vi "控制箱到引脚映射.vi"(1 "导通控制箱":string) -> (0 "导通引脚":string)   [LabVIEW 2020]
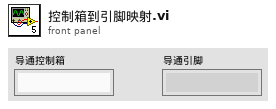
[diagram p1: front panel]
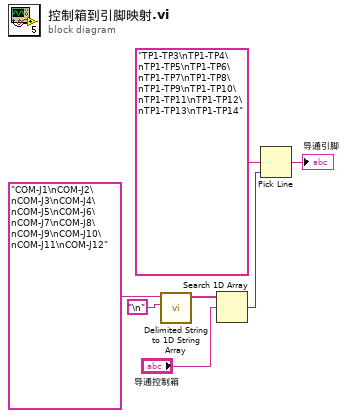
[diagram p0: block diagram]
diagram:
  n1 = call <vilib>:"Delimited String to 1D String Array.vi"("delimiter"="\n", "delimited string"="COM-J1\nCOM-J2\nCOM-J3\nCOM-J4\nCOM-J5\nCOM-J6\nCOM-J7\nCOM-J8\nCOM-J9\nCOM-J10\nCOM-J11\nCOM-J12") -> ("string array"=w3:string[])  [unwired: 9 in]
  n2 = Search 1D Array(1D array=w3, element="导通控制箱") -> (index of element=w1:i32)  [unwired: 1 in]
  n3 = Pick Line(multi-line string="TP1-TP3\nTP1-TP4\nTP1-TP5\nTP1-TP6\nTP1-TP7\nTP1-TP8\nTP1-TP9\nTP1-TP10\nTP1-TP11\nTP1-TP12\nTP1-TP13\nTP1-TP14", line index=w1) -> (output string=→"导通引脚":string)  [unwired: 1 in]
